vi "saveToFile.vi"(9 "SigJSONbuffer":string, 10 "dimensions":i64[](array[numeric]), 11 "String":string) -> (0 "error out":errorcluster)   [LabVIEW 2014]
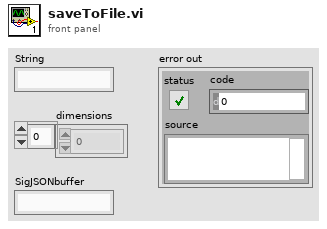
[diagram p1: front panel]
types:
  T1 = enum16{"open", "replace", "create", "open or create", "replace or create", "replace or create with confirmation"}
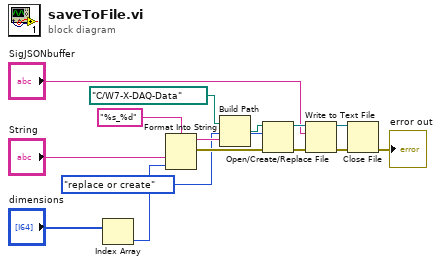
[diagram p0: block diagram]
diagram:
  n1 = Index Array(array="dimensions") -> (element=w13:i64)  [unwired: 1 in]
  n2 = Format Into String(format string="%s_%d", "String", w13) -> (resulting string=w15:string, error out=w14:errorcluster)  [unwired: 2 in]
  n3 = Build Path(base path=path "C:/W7-X-DAQ-Data", name or relative path=w15) -> (appended path=w10:path)
  n4 = Open/Create/Replace File(file path (use dialog)=w10, error in=w14, operation (0:open)=T1."replace or create") -> (refnum out=w8:refnum<file>, error out=w9:errorcluster)  [unwired: 3 in, 1 out]
  n5 = Write to Text File(file (use dialog)=w8, text="SigJSONbuffer", error in=w9) -> (refnum out=w7:refnum<file>, error out=w5:errorcluster)  [unwired: 1 in, 1 out]
  n6 = Close File(refnum=w7, error in=w5) -> (error out=→"error out":errorcluster)  [unwired: 1 out]
